vi "On Status Bar Text Changed.vi"(8 "error in (no error)":errorcluster, 10 "Text":string, 11 "WebView2 Event Filter Interface in":refnum<class "WebView2 Event Filter Interface.lvclass">) -> (0 "error out":errorcluster)   [LabVIEW 2025, in "WebView2.lvlib" / "WebView2 Event Filter Interface.lvclass"]
uses:
  WebView2 Event Filter Interface.lvclass
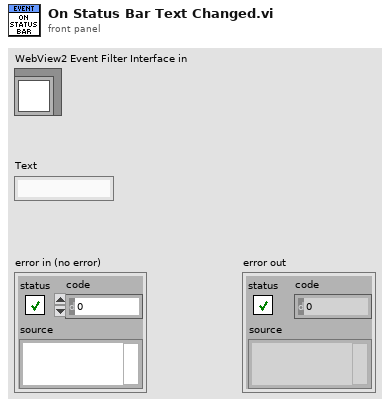
[diagram p1: front panel]
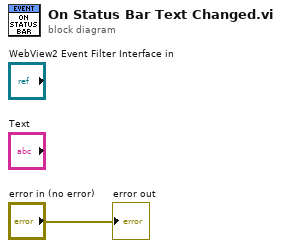
[diagram p0: block diagram]
diagram:
  "error out" <- "error in (no error)"
